vi "SLL DE Create DAQmx task for given channels ver 1.vi"(7 "Channel Type":T1, 8 "error in (no error)":errorcluster, 10 "Channel Array":cluster{"Device Channel List":string[]}[](array[cluster]), 11 "Devices Names":string[](array[string])) -> (0 "error out":errorcluster, 3 "Array of Tasks":refnum<k21>[](array[refnum]))   [LabVIEW 2013]
doc: "Copyright © 2005, Soliton Technologies.\nAll rights reserved."
uses:
  Controls/SLL DE DAQ Engine Channel Types.ctl
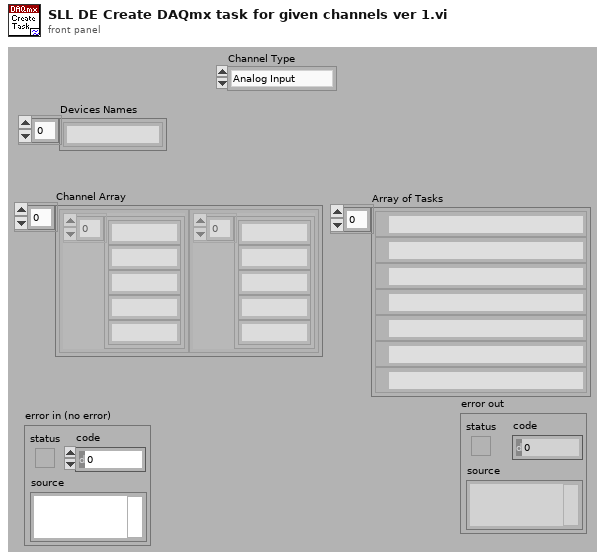
[diagram p1: front panel]
types:
  T1 = typedef "SLL DE DAQ Engine Channel Types.ctl" = enum16{"Analog Input", "Analog Output", "Digital Input", "Digital Output"}
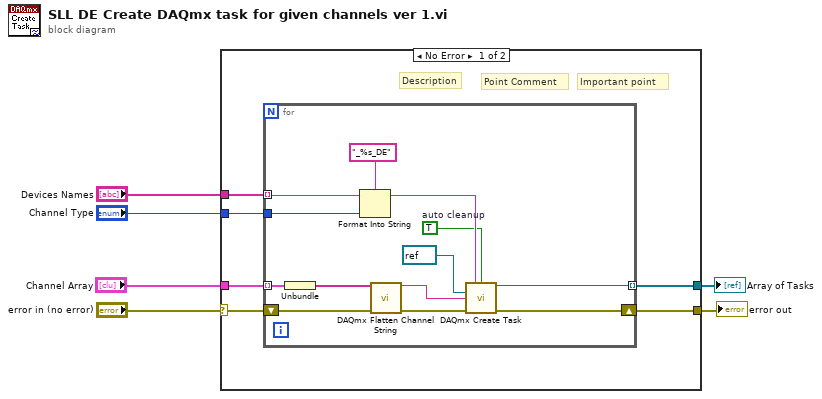
[diagram p0: block diagram]
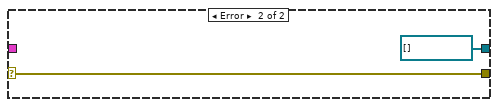
[diagram p2: hidden frame]
diagram:
  n1 = case shown="No Error" "error in (no error)" {
    selector: "error in (no error)" -> [w10 w27]
    tunnel: [w9 w27] -> w5
    tunnel: "Channel Type" -> [w12 _]
    tunnel: [w11 refnum<k21>[] []] -> w3
    tunnel: "Devices Names" -> [w8 _]
    tunnel: "Channel Array" -> [w7 _]
    frame No Error {
      # "Point Comment"
      # "Important point"
      # "Description"
      n2 = for {
        shift-right: [w20] -> w9
        shift-left: w10 -> [w24]
        tunnel: w12 -> [w22]
        tunnel: [w16] -> w11 mode=indexing
        tunnel: w8 -> [w15] mode=indexing
        tunnel: w7 -> [w14] mode=indexing
        w18 = TRUE  # auto cleanup
        n3 = Unbundle(w14) -> ("Device Channel List"=w13:string[])
        n4 = Format Into String(format string="_%s_DE", initial string=w15, w22) -> (resulting string=w19:string)  [unwired: 1 in, 1 out]
        n5 = call <vilib>:"DAQmx Flatten Channel String.vi"("names in"=w13, "error in"=w24) -> ("names out"=w25:string, "error out"=w23:errorcluster)  [unwired: 12 in]
        n6 = call <vilib>:"DAQmx Create Task.vi"("new task name"=w19, "auto cleanup"=w18, "task to copy"=refnum<k21> refnum, "global virtual channels"=w25, "error in"=w23) -> ("task out"=w16:refnum<k21>, "error out"=w20:errorcluster)  [unwired: 9 in]
      }
    }
    frame Error {
    }
  }
  "error out" <- w5
  "Array of Tasks" <- w3
